vi "Unload.vi"(8 "error in":errorcluster, 11 "PickupTool in":refnum<class "PickerTool Class.lvclass">) -> (0 "error out":errorcluster, 3 "Gantry out":refnum<class "Gantry Class.lvclass">)   [LabVIEW 2011, in "PickerTool Class.lvclass"]
uses:
  PickerTool Class.lvclass
  Gantry Class/Gantry Class.lvclass
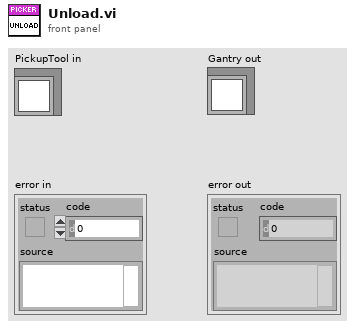
[diagram p1: front panel]
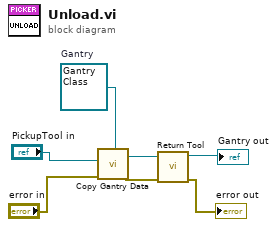
[diagram p0: block diagram]
diagram:
  w5 = refnum<class "Gantry Class.lvclass"> refnum  # Gantry
  n1 = call "Copy Gantry Data.vi"("error in"="error in", "Gantry Source"="PickupTool in", "Gantry Dest"=w5) -> ("error out"=w6:errorcluster, "Gantry Result"=w7:refnum<class "Gantry Class.lvclass">)  [unwired: 7 in]
  n2 = call-dynamic "Return Tool.vi"("error in"=w6, "Gantry in"=w7) -> ("error out"=→"error out":errorcluster, "Gantry out"=→"Gantry out":refnum<class "Gantry Class.lvclass">)  [unwired: 8 in]
